vi "FGV_MIDASHandlingTime.vi"(0 "Midas Handling Time":dbl, 4 "Enum":enum16{"Set", "GetLast", "GetAverage"}(ring)) -> (5 "Midas Handling Time":dbl)   [LabVIEW 2018]
panel:
  out "Array Index":i32
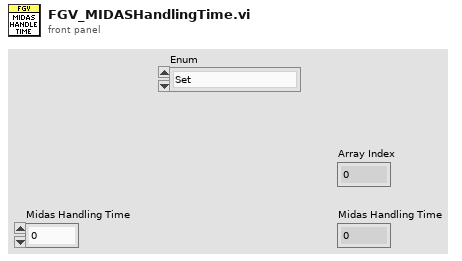
[diagram p1: front panel]
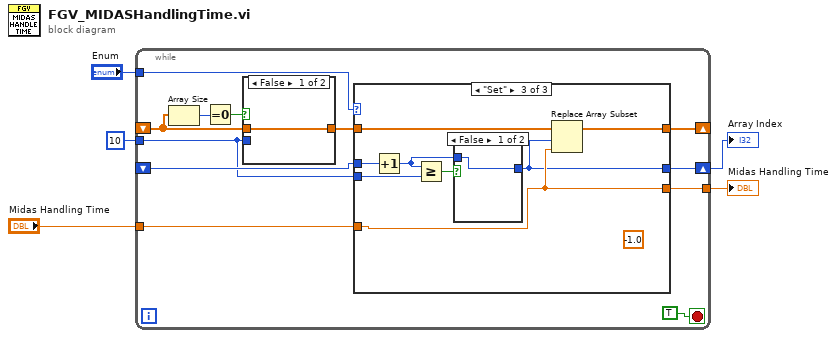
[diagram p0: block diagram]
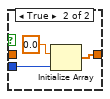
[diagram p2: hidden frame]
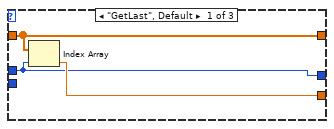
[diagram p3: hidden frame]
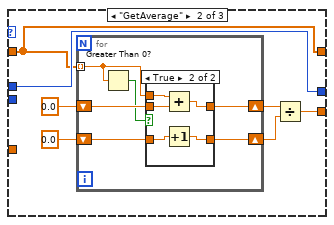
[diagram p4: hidden frame]
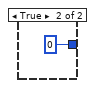
[diagram p6: hidden frame]
diagram:
  n1 = while {
    shift-right: [w17] -> _
    shift-left: _ -> [w9]
    tunnel: "Midas Handling Time" -> [w15]
    tunnel: [w16] -> w3
    tunnel: "Enum" -> [w14]
    shift-right: [w11] -> w1
    shift-left: _ -> [w12]
    tunnel: 10 ("dimension size") -> [w6]
    stop <- TRUE stop-if-true
    n2 = Array Size(array=w9) -> (size(s)=w8:i32)
    n3 = Equal To 0?(x=w8) -> (x = 0?=w7:bool)
    n4 = case shown="False" w7 {
      tunnel: [w18 w20] -> w10
      tunnel: w9 -> [w18 _]
      tunnel: w6 -> [_ w19]
      frame False {
      }
      frame True {
        n5 = Initialize Array(0.0 ("element"), w19) -> (w20:dbl[])
      }
    }
    n6 = case shown="\"Set\"" w14 {
      tunnel: [w23 w25 w49] -> w16
      tunnel: [w24 w29 w51] -> w17
      tunnel: w10 -> [w24 w29 w48]
      tunnel: w15 -> [_ _ w49]
      tunnel: w12 -> [w22 w30 w50]
      tunnel: [w22 w30 w45] -> w11
      tunnel: w6 -> [_ _ w47]
      frame "GetLast", Default {
        n7 = Index Array(array=w24, index=w22) -> (element=w23:dbl)
      }
      frame "GetAverage" {
        n8 = for {
          shift-right: [w37] -> w31
          shift-left: 0.0 -> [w36]
          tunnel: w29 -> [w35] mode=indexing
          shift-right: [w33] -> w28
          shift-left: 0.0 -> [w32]
          n9 = Greater Than 0?(x=w35) -> (x > 0?=w34:bool)
          n10 = case shown="True" w34 {
            tunnel: [w38 w44] -> w37
            tunnel: w36 -> [w38 w43]
            tunnel: w35 -> [_ w42]
            tunnel: [w39 w41] -> w33
            tunnel: w32 -> [w39 w40]
            frame False {
            }
            frame True {
              n11 = Add(x=w42, y=w43) -> (x+y=w44:dbl)
              n12 = Increment(x=w40) -> (x+1=w41:dbl)
            }
          }
        }
        n13 = Divide(x=w31, y=w28) -> (x/y=w25:dbl)
      }
      frame "Set" {
        (unwired) -1.0
        n14 = Increment(x=w50) -> (x+1=w46:i32)
        n15 = Greater Or Equal?(x=w46, y=w47) -> (x >= y?=w52:bool)
        n16 = case shown="False" w52 {
          tunnel: [w53 0] -> w45
          tunnel: w46 -> [w53 _]
          frame False {
          }
          frame True {
          }
        }
        n17 = Replace Array Subset(array=w48, new element=w49, index=w45) -> (w51:dbl[])
      }
    }
  }
  "Midas Handling Time" <- w3
  "Array Index" <- w1
